vi "test_sicm_main.vi"() -> ()   [LabVIEW 2016]
uses:
  <vilib>/rvi/DesktopExecutionNode/Execution/niFpgaDEN_Execute.vi
  <vilib>/rvi/DesktopExecutionNode/DesktopExecutionNode.xnode
panel:
  in  "enablethicks1":i32=2000
  out "debug":T1(array[cluster])
  out "Trigger":T2(array[cluster])
  in  "enablethicks":i32=2000
  out "current":dbl[](graph)
  out "Progress":dbl(slide) scale=0.0..1.0
  out "height":dbl[](graph)
  out "sicm.o.height":fxp<+/-,22,4>
  in  "sicm.i.current":T3
  in  "sicm.p.modes":T4={"sicm.p.enable"=FALSE, "sicm.p.adaptiveStepDown"=FALSE, "sicm.p.relSetpoint"=TRUE}
  in  "sicm.p.params":T5={"sicm.p.setPoint"=0.8999996185302734, "stepDown"=-0.04000002145767212, "retractHeight"=0.10000002384185791, "adaptiveMin"=0.0}
  in  "sicm.p.clocks":T6={"inverseDecimation"=0.0, "decimation"=2, "waveSize"=128, "pixelDecimation"=0}
  in  "sicm.blc.p.params":T7={"se.blc.p.postRetractDelay"=150, "se.blc.p.windowSize"=10, "se.blc.p.updateFactor"=-8}
  in  "d0":dbl=0.3
  in  "D":dbl=0.001
  in  "Idc":dbl=5000.0
  in  "Simulation ticks":i32=10000
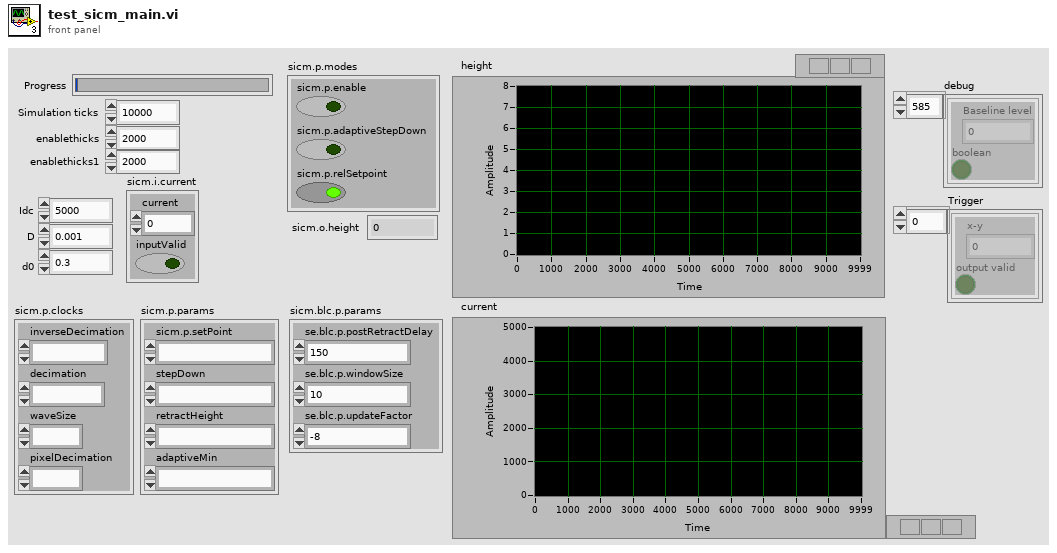
[diagram p1: front panel]
types:
  T1 = cluster{"Baseline level":fxp<+/-,22,21>, "boolean":bool}[]
  T2 = cluster{"x-y":fxp<+/-,22,4>, "output valid":bool}[]
  T3 = cluster{"current":fxp<+/-,24,16>, "inputValid":bool}
  T4 = cluster{"sicm.p.enable":bool, "sicm.p.adaptiveStepDown":bool, "sicm.p.relSetpoint":bool}
  T5 = cluster{"sicm.p.setPoint":fxp<+,20,0>, "stepDown":fxp<+/-,28,4>, "retractHeight":fxp<+/-,28,4>, "adaptiveMin":fxp<+,10,0>}
  T6 = cluster{"inverseDecimation":fxp<+,22,0>, "decimation":u16, "waveSize":u16, "pixelDecimation":u16}
  T7 = cluster{"se.blc.p.postRetractDelay":u16, "se.blc.p.windowSize":u16, "se.blc.p.updateFactor":i16}
  T8 = cluster{"x-y":fxp<+/-,22,4>, "output valid":bool}
  T9 = cluster{"Baseline level":fxp<+/-,22,21>, "boolean":bool}
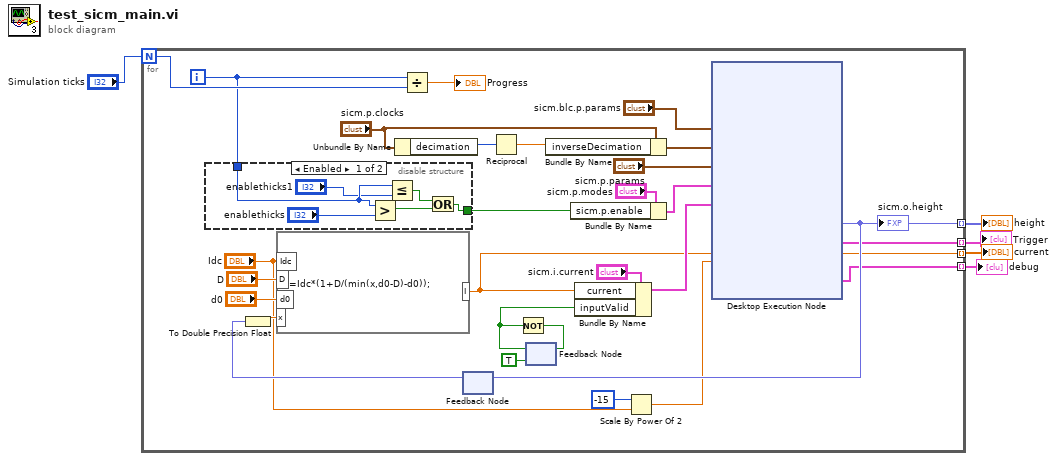
[diagram p0: block diagram]
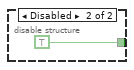
[diagram p2: hidden frame]
diagram:
  n1 = for {
    N: "Simulation ticks" -> [w29]
    tunnel: [w25] -> w4 mode=indexing
    tunnel: [w14] -> w3 mode=indexing
    tunnel: [w10] -> w2 mode=indexing
    tunnel: [w9] -> w1 mode=indexing
    i -> [w12]
    n2 = disable-structure shown="Enabled" {
      disable-tunnel: w12 -> [w35 _]
      disable-tunnel: [w36 TRUE] -> w11
      frame Enabled {
        n3 = Greater?(x=w35, y="enablethicks") -> (0:w37:bool)
        n4 = Less Or Equal?(x=w35, y="enablethicks1") -> (x <= y?=w38:bool)
        n5 = Or(x=w38, y=w37) -> (x .or. y?=w36:bool)
      }
      frame Disabled {
      }
    }
    n6 = Unbundle By Name("sicm.p.clocks") -> ("decimation"=w15:u16)
    n7 = Divide(x=w12, y=w29) -> (x/y=→"Progress":dbl)
    n8 = feedback #1() -> (w24:fxp<+/-,22,4>)  [unwired: 1 in]
    n9 = To Double Precision Float(number=w24) -> (double precision float=w23:dbl)
    n10 = formula code="I=Idc*(1+D/(min(x,d0-D)-d0));"("Idc"="Idc", "D"="D", "d0"="d0", "x"=w23) -> ("I"=w14:dbl)
    n11 = Reciprocal(x=w15) -> (1/x=w16:dbl)
    n12 = feedback #2(TRUE) -> (w19:bool)
    n13 = Not(x=w19) -> (.not. x?=w21:bool)
    n14 = feedback-in #2(w21) -> ()
    n15 = Bundle By Name(cluster="sicm.p.clocks", "inverseDecimation"=w16) -> (w18:T6)
    n16 = Bundle By Name(cluster="sicm.p.modes", "sicm.p.enable"=w11) -> (w13:T4)
    n17 = Bundle By Name(cluster="sicm.i.current", "current"=w14, "inputValid"=w19) -> (w22:T3)
    n18 = Scale By Power Of 2(n=i16 -15, x="Idc") -> (x*2^n=w7:dbl)
    n19 = xnode "Desktop Execution Node"("sicm.blc.p.params"="sicm.blc.p.params", "sicm.p.clocks"=w18, "sicm.p.params"="sicm.p.params", "sicm.p.modes"=w13, "sicm.i.current"=w22, "baseline"=w7) -> ("sicm.o.height"=w25:fxp<+/-,22,4>, "sicm.triggerHeight"=w10:T8, "debug"=w9:T9)  [unwired: 1 in, 1 out]
    "sicm.o.height" <- w25
    n20 = feedback-in #1(w25) -> ()
  }
  "height" <- w4
  "current" <- w3
  "Trigger" <- w2
  "debug" <- w1
